vi "Pot Modules.vi"(8 "error in":errorcluster, 11 "Potting Procedure in":refnum<class "Potting Procedure.lvclass">) -> (0 "error out":errorcluster, 3 "Potting Procedure out":refnum<class "Potting Procedure.lvclass">)   [LabVIEW 2011, in "Potting Procedure.lvclass"]
uses:
  Potting Procedure.lvclass
  Shared Components/SyringeTool Class/SyringeTool Class.lvclass
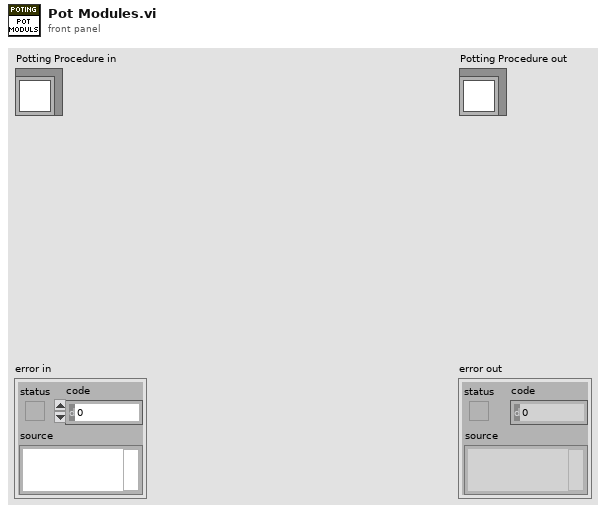
[diagram p1: front panel]
types:
  T1 = typedef "Module Potting Data.ctl" = cluster{"HDI Bond Pad Groups":T2[], "BBM Bond Pad Groups":T2[], "TBM - TBM Side":T2[], "TBM - HDI Side":T2[], "Address Pads":T2[], "Chuck":i32, "Slot":i32, "HV Points":refnum<class "Vec3d Class.lvclass">[]}
  T2 = typedef "3d Line.ctl" = cluster{"Start":refnum<class "Vec3d Class.lvclass">, "End":refnum<class "Vec3d Class.lvclass">}
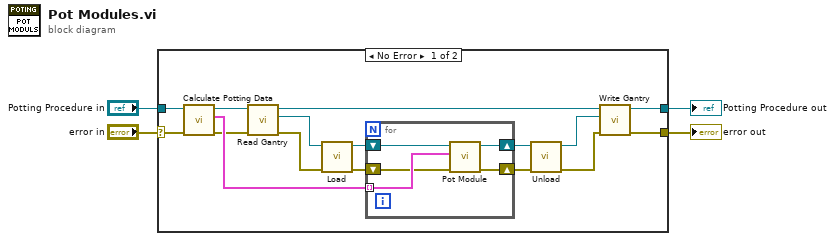
[diagram p0: block diagram]
diagram:
  n1 = case shown="No Error" "error in" {
    selector: "error in" -> [w6 w27]
    tunnel: [w5 w27] -> w3
    tunnel: [w7 w26] -> w1
    tunnel: "Potting Procedure in" -> [w20 w26]
    frame No Error {
      n2 = call "Calculate Potting Data.vi"("error in"=w6, "Potting Procedure in"=w20) -> ("error out"=w15:errorcluster, "Module Potting Data"=w19:T1[], "Potting Procedure out"=w18:refnum<class "Potting Procedure.lvclass">)  [unwired: 7 in]
      n3 = call-dynamic "Read Gantry.vi"("error in (no error)"=w15, "Potting Procedure in"=w18) -> ("error out"=w14:errorcluster, "Gantry"=w17:refnum<class "Gantry Class.lvclass">, "Potting Procedure out"=w11:refnum<class "Potting Procedure.lvclass">)  [unwired: 7 in]
      n4 = call "Load.vi"("error in"=w14, "Gantry in"=w17) -> ("error out"=w13:errorcluster, "SyringeTool out"=w16:refnum<class "SyringeTool Class.lvclass">)  [unwired: 8 in]
      n5 = for {
        tunnel: w19 -> [w25] mode=indexing
        shift-right: [w22] -> w12
        shift-left: w16 -> [w23]
        shift-right: [w21] -> w9
        shift-left: w13 -> [w24]
        n6 = call "Pot Module.vi"("error in"=w24, "Module Potting Data"=w25, "SyringeTool in"=w23) -> ("error out"=w21:errorcluster, "SyringeTool out"=w22:refnum<class "SyringeTool Class.lvclass">)  [unwired: 7 in]
      }
      n7 = call "Unload.vi"("error in"=w9, "SyringeTool in"=w12) -> ("error out"=w8:errorcluster, "Gantry out"=w10:refnum<class "Gantry Class.lvclass">)  [unwired: 8 in]
      n8 = call-dynamic "Write Gantry.vi"("error in (no error)"=w8, "Gantry"=w10, "Potting Procedure in"=w11) -> ("error out"=w5:errorcluster, "Potting Procedure out"=w7:refnum<class "Potting Procedure.lvclass">)  [unwired: 7 in]
    }
    frame Error {
    }
  }
  "error out" <- w3
  "Potting Procedure out" <- w1
